vi "read_timing_array.vi"(4 "error in":errorcluster, 5 "input array":dbl[](array[numeric]), 6 "time unit":enum16{"s", "ms", "us", "ns"}(ring), 7 "VISA resource in":refnum<visa-resource-name>) -> (0 "error out 2":errorcluster, 1 "delay array":dbl[](array[numeric]), 3 "VISA resource out":refnum<visa-resource-name>)   [LabVIEW 2011]
doc: "Reads all delay values stored in the DG645 and returns them in an array, from t0 to H.\nSee DG645 documentation for mor info."
panel:
  in  "bytes to read":u32=256
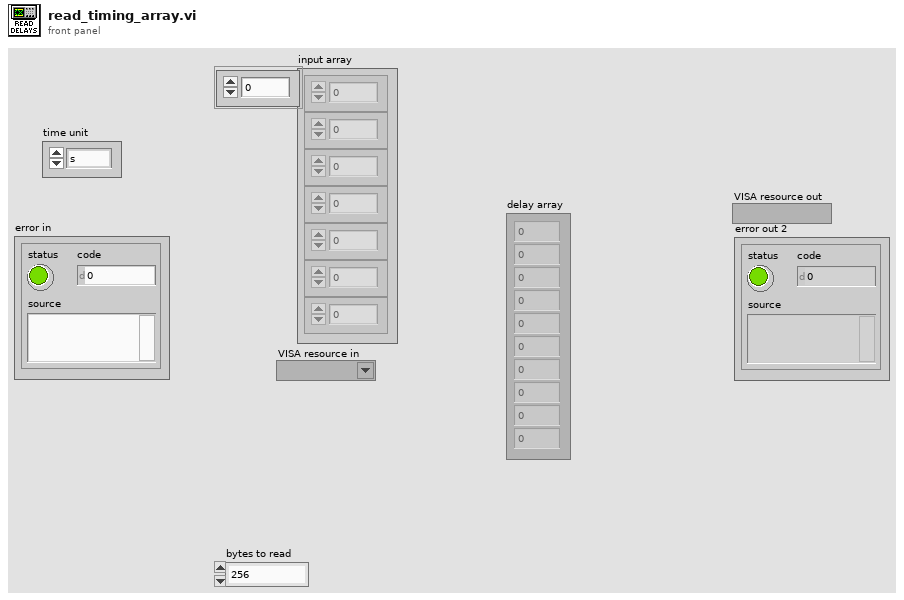
[diagram p1: front panel]
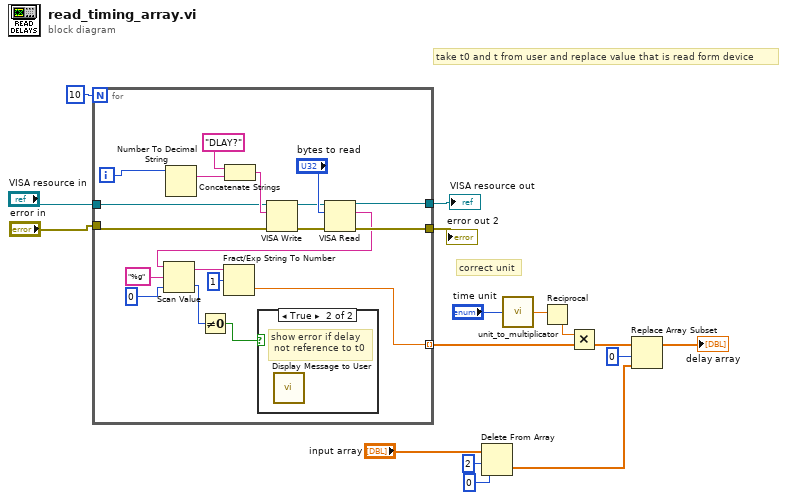
[diagram p0: block diagram]
diagram:
  # "correct unit"
  # "take t0 and t from user and replace value that is read form device"
  n1 = for {
    N: 10 -> [_]
    tunnel: "error in" -> [w32]
    tunnel: [w29] -> w9 mode=indexing
    tunnel: [w26] -> w12
    tunnel: "VISA resource in" -> [w21]
    tunnel: [w20] -> w13
    i -> [w17]
    n2 = Number To Decimal String(number=w17) -> (decimal integer string=w28:string)  [unwired: 1 in]
    n3 = Concatenate Strings("DLAY?" ("string"), w28) -> (w27:string)
    n4 = VISA Write(VISA resource name=w21, write buffer=w27, error in (no error)=w32) -> (VISA resource name out=w34:refnum<visa-resource-name>, error out=w33:errorcluster)  [unwired: 1 out]
    n5 = VISA Read(VISA resource name=w34, byte count="bytes to read", error in (no error)=w33) -> (VISA resource name out=w20:refnum<visa-resource-name>, read buffer=w19:string, error out=w26:errorcluster)  [unwired: 1 out]
    n6 = Scan Value(string=w19, format string="%g", default (0 dbl)=u16 0) -> (output string=w23:string, value=w22:u16)
    n7 = Not Equal To 0?(x=w22) -> (x != 0?=w18:bool)
    n8 = Fract/Exp String To Number(string=w23, offset=1) -> (number=w29:dbl)  [unwired: 2 in, 1 out]
    n9 = case shown="True" w18 {
      frame False {
      }
      frame True {
        # "show error if delay\n not reference to t0"
        n10 = call "Display Message to User"() -> ()  [unwired: 10 in, 2 out]
      }
    }
  }
  "VISA resource out" <- w13
  "error out 2" <- w12
  n11 = Delete From Array(array="input array", length=2, index=0) -> (deleted portion=w5:dbl[])  [unwired: 1 out]
  n12 = call "unit_to_multiplicator.vi"("time unit"="time unit") -> ("multiplicator"=w2:dbl)
  n13 = Reciprocal(x=w2) -> (1/x=w1:dbl)
  n14 = Multiply(x=w1, y=w9) -> (x*y=w3:dbl[])
  n15 = Replace Array Subset(array=w3, new element=w5, index=0) -> (→"delay array":dbl[])
